vi "NV measurements.vi"(0 "Number of samples":dbl=50000.0, 1 "Pulse mode":T1(ring), 2 "Initial duration (ns)":dbl=1.0 format="%#_13g", 3 "Final duration (ns)":dbl=1.0 format="%#_13g", 4 "AOM on":dbl[unit]=9.999999999999999e-06 format="%#_13p", 5 "AOM off":dbl[unit]=9.999999999999999e-05 format="%#_13p", 6 "N type output level value (-136dBm to 0 dBm)":dbl=-20.0, 7 "Duration increment (ns)":dbl=1.0 format="%#_13g", 8 "file (use dialog)":path=path "C:/Users/Choi group/Dropbox/Labbook/Quantum Optics/hBN/230726/attoDRY", 9 "pi":dbl[unit] format="%#_13p", 10 "Initial frequency (MHz)":dbl=1500.0 format="%#_13g", 11 "pi/2":dbl[unit] format="%#_13p", 12 "Final frequency (MHz)":dbl=2500.0 format="%#_13g", 13 "Contrast calculation":T3(ring), 14 "Frequency increment (MHz)":dbl=10.0 format="%#_13g", 15 "Modulation type":u16(ring)=4 items=["AM/ASK"=0, "FM/FSK"=1, "PM/PSK"=2, "Sweep"=3, "Pulse"=4, "Blank"=5, "QAM"=7, "CPM"=8, "VSB"=9], 16 "Measurement #":i32=11, 18 "Averaging?":bool, 19 "Parameters logging?":bool=TRUE) -> ()   [LabVIEW 2015]
uses:
  Libraries/Stanford Research SG39x Series/Stanford Research SG39x Series.lvlib
  <vilib>/Utility/file.llb/Write Delimited Spreadsheet (string).vi
  Libraries/SR400/Public/Typedefs/Output Scale.ctl
  Libraries/SR400/SR400.lvlib
panel:
  in  "file path for measurement parameters":path=path "C:/Users/Choi group/Dropbox/Labbook/Quantum Optics/hBN/230726/attoDRY/parameters log.txt"
  out "file?":bool
  in  "Tab Control":T2(tab)=enum."AFG3252"
  in  "VISA_SG396":refnum<visa-resource-name>="GPIB0::27::INSTR"
  in  "Location of spinapi.dll":path=path "C:/SpinCore/SpinAPI/lib/spinapi64.dll"
  in  "pi_Y":dbl[unit] format="%#_13p"
  in  "VISA_SR400_1":refnum<visa-resource-name>="GPIB0::18::INSTR"
  in  "VISA_SR400_2":refnum<visa-resource-name>="GPIB0::18::INSTR"
  in  "Gate A width":dbl[unit]=8.000000000000001e-06
  in  "Gate A delay":dbl[unit]=2.0000000000000003e-06
  in  "Gate B width":dbl[unit]=8.000000000000001e-06
  in  "Gate B delay":dbl[unit]=2.0000000000000003e-06
  in  "Gate delay offset":dbl[unit]=7.000000000000001e-09
  in  "Gate width offset":dbl[unit]=8e-09
  in  "Gain":dbl=0.6
  in  "margin (ns)":i32=20
  in  "resolution (ns)":dbl=0.5 format="%#_13g"
  in  "AFG to MW switch delay":dbl[unit]=2.3000000000000002e-07 format="%#_13g"
  in  "N of XY8-N":i32=1
  in  "MW switch margin (ns)":dbl=30.0 format="%#_13g"
  out "Current frequency (MHz)":dbl=2980.0 format="%#.9f"
  out "Contrast":dbl=0.9066760283189983
  out "Sig1_temp":dbl=15496.0
  out "Sig2_temp":dbl=17091.0
  out "Ref1_temp":dbl=15202.0
  out "Ref2_temp":dbl=17166.0
  out "Iteration":i32=1662
  out "Current duration":dbl[unit]
  out "Averaged counts":dbl=0.9066760283189983
  out "XY Graph":cluster{"Y":dbl[], "Y":dbl[]}[](graph)=[{"Y"=[10.0, 12.0, 14.0, 16.0, 18.0, 20.0, 22.0, 24.0, 26.0, 28.0, 30.0, 32.0, 34.0, 36.0, 38.0, 40.0, 42.0, 44.0, 46.0, 48.0, 50.0, 52.0, 54.0, 56.0, 58.0, 60.0, 62.0, 64.0, 66.0, 68.0, 70.0, 72.0, 74.0, 76.0, 78.0, 80.0, 82.0, 84.0, 86.0, 88.0, 90.0, 92.0, 94.0, 96.0, 98.0, 100.0], "Y"=[0.8767203858369602, 0.8691455977263308, 0.8745225141798818, 0.9030268088786394, 0.9378455450154222, 0.9275370747310265, 0.9308731504766361, 0.9057829759584146, 0.8666319504715616, 0.8803564101061023, 0.906591799730947, 0.9180885370858985, 0.9439413797211962, 0.9016052661970204, 0.8839480638860162, 0.8758135750813575, 0.8816878889967453, 0.913326362263274, 0.9088317463937511, 0.9162288551469315, 0.9055664853604907, 0.9089218250508573, 0.8930382664822499, 0.8875780707841776, 0.9212244897959184, 0.9054543364561183, 0.8933922728055571, 0.9381969714755253, 0.8942631517826036, 0.8838066088533696, 0.8963005448809865, 0.9031774407473616, 0.9180577520060914, 0.9075721912853779, 0.8828040674884963, 0.90195394277739, 0.8791781135531136, 0.9186380980334605, 0.9048862581244196, 0.9063314603487227, 0.9013971137814063, 0.8959866605335787, 0.9040195451108138, 0.8972309118294519, 0.9009098914000586, 0.9066760283189983]}]
  out "XY Graph 2":cluster{"Y":dbl[], "Y":dbl[]}[](graph)=[{"Y"=[2980.0], "Y"=[0.8767203858369602]}]
  in  "stop":bool
  out "file":refnum<file>
  # "IQ modulation ON: QAM\nIQ modulation OFF: Pulse"
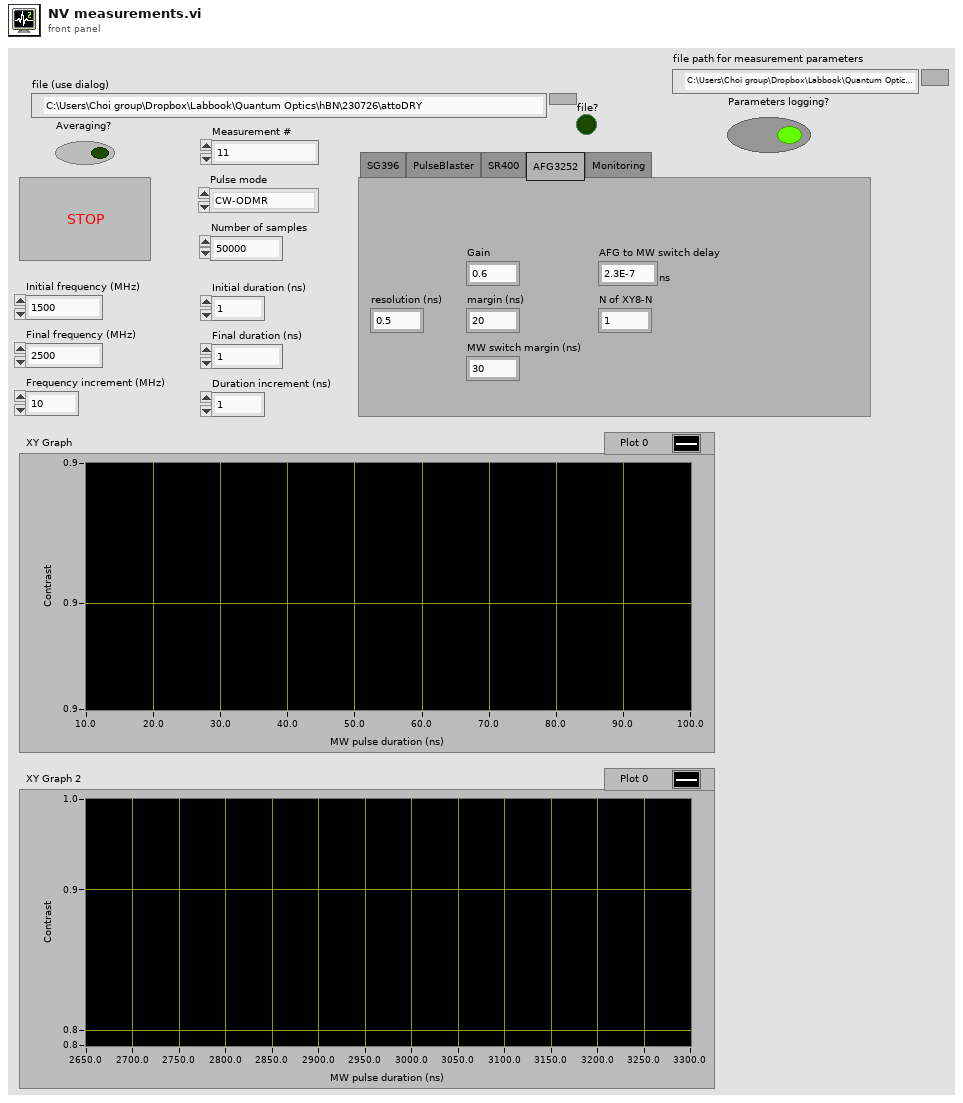
[diagram p1: front panel]
types:
  T1 = enum16{"CW-ODMR", "Rabi", "Rabi_IQ", "Ramsey", "Spin echo decay", "Spin echo_IQ", "CPMG", "XY4", "XY8", "XY8-N", "Corr-XY8", "T1 relaxation", "T1_IQ"}
  T2 = enum32{"SG396", "PulseBlaster", "SR400", "AFG3252", "Monitoring"}
  T3 = enum16{"sig1/sig2", "sig1/ref2", "(sig2-sig1)/(sig2+sig1)", "(sig2-sig1)/ref1"}
  T4 = enum16{"open", "replace", "create", "open or create", "replace or create", "replace or create with confirmation"}
  T5 = typedef "SR400.lvlib/Output Scale.ctl" = enum16{"Log", "987######", "#876#####", "##765####", "###654###", "####543##", "#####432#", "######321"}
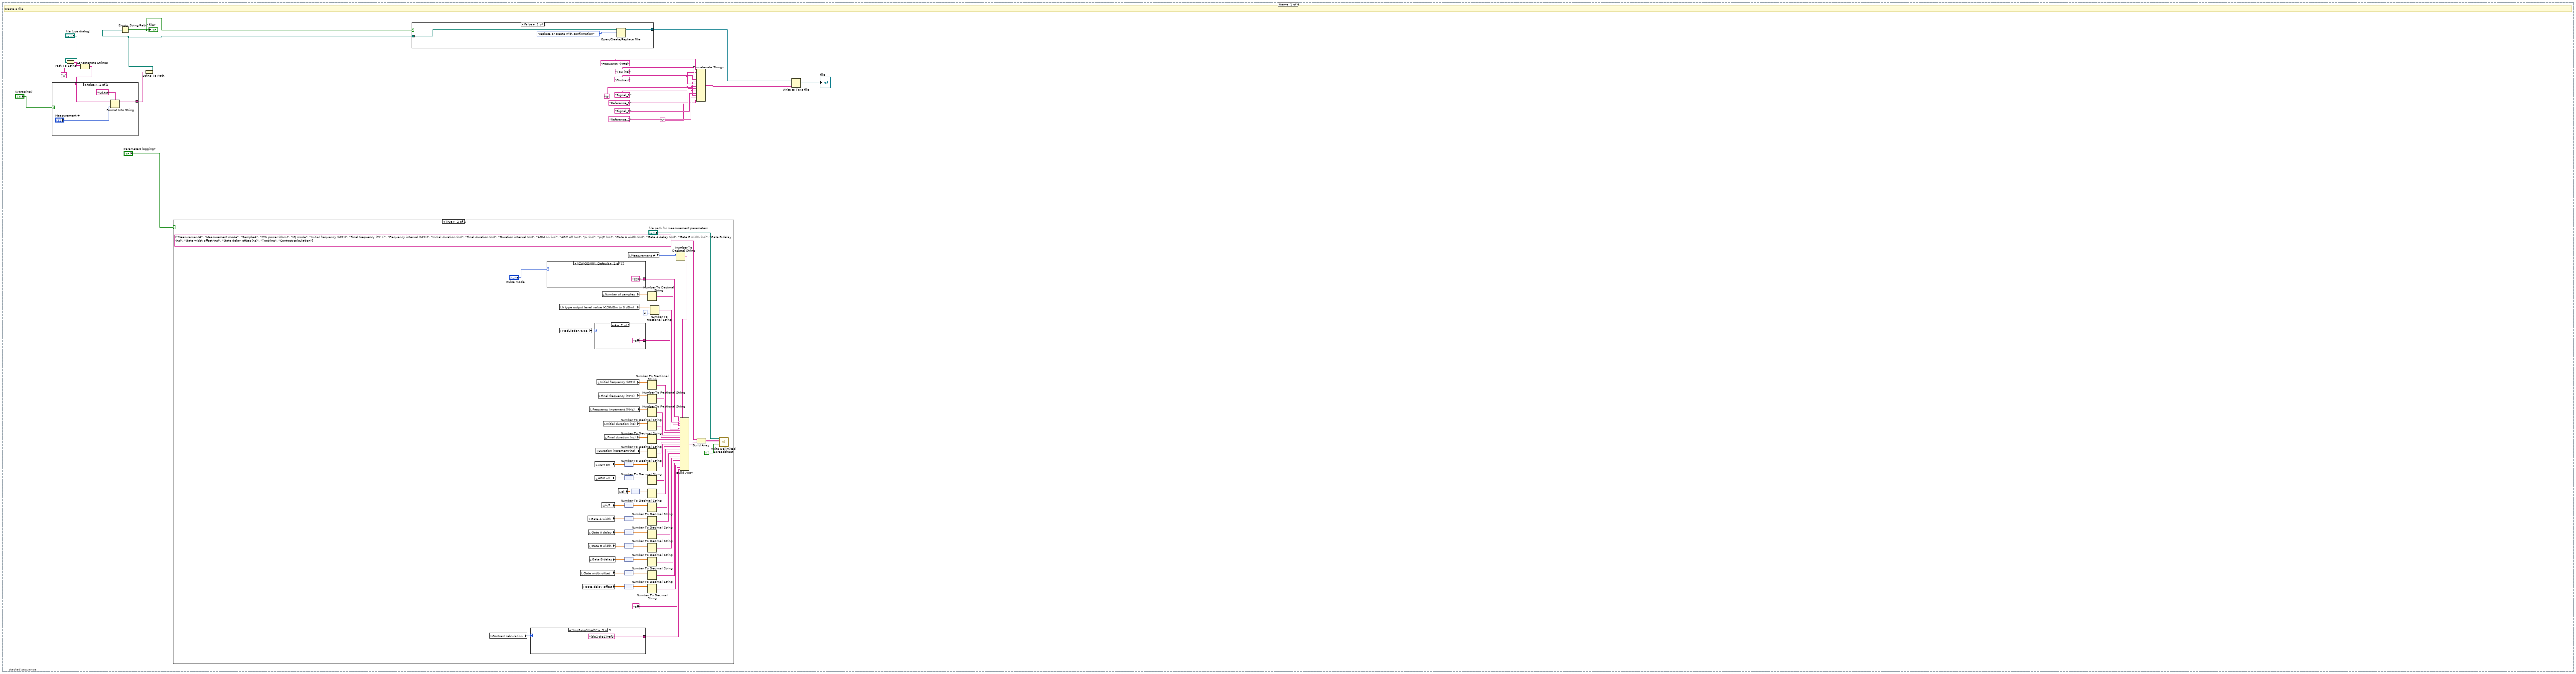
[diagram p2: hidden frame]
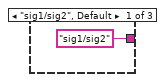
[diagram p5: hidden frame]
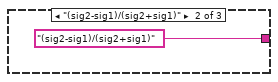
[diagram p6: hidden frame]
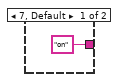
[diagram p7: hidden frame]
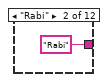
[diagram p8: hidden frame]
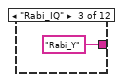
[diagram p9: hidden frame]
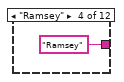
[diagram p10: hidden frame]
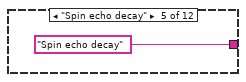
[diagram p11: hidden frame]
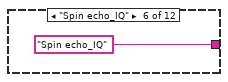
[diagram p12: hidden frame]
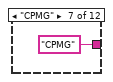
[diagram p13: hidden frame]
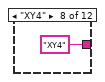
[diagram p14: hidden frame]
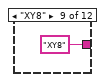
[diagram p15: hidden frame]
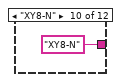
[diagram p16: hidden frame]
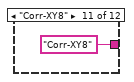
[diagram p17: hidden frame]
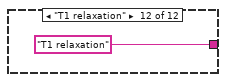
[diagram p18: hidden frame]
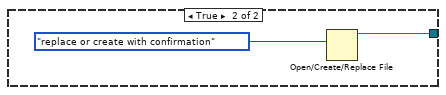
[diagram p19: hidden frame]
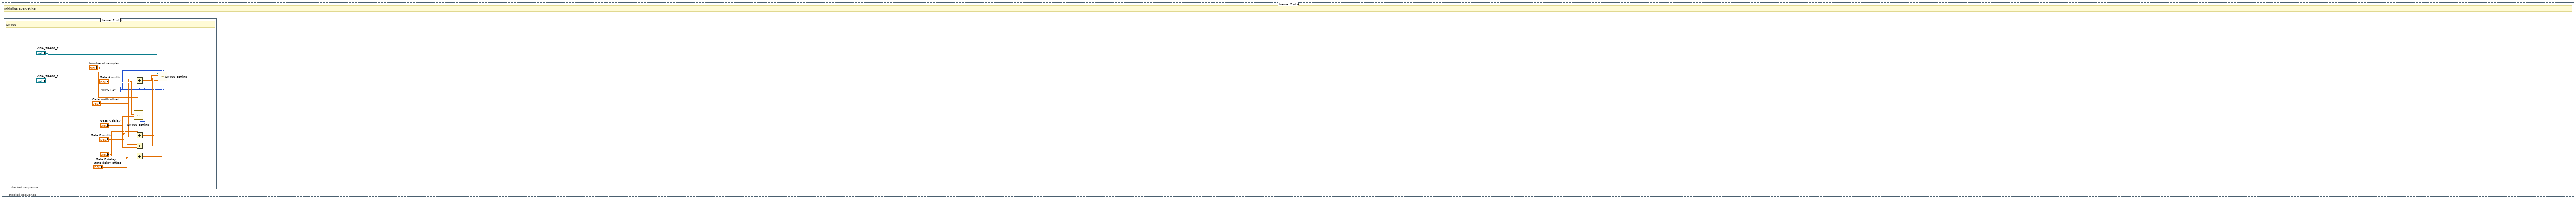
[diagram p20: hidden frame]
diagram:
  n1 = stacked-sequence {
    frame #0 {
      w1 = "\t"
      # "Create a file"
      n2 = Path To String(path="file (use dialog)") -> (string=w6:string)
      n3 = Concatenate Strings(w6, "\\" ("string")) -> (w4:string)
      n4 = case shown="False" "Averaging?" {
        tunnel: w4 -> [w23 w26]
        tunnel: [w24 w26] -> w7
        frame False {
          n5 = Format Into String(format string="%d.txt", initial string=w23, "Measurement #") -> (resulting string=w24:string)  [unwired: 1 in, 1 out]
        }
        frame True {
        }
      }
      n6 = String To Path(string=w7) -> (path=w3:path)
      n7 = Empty String/Path?(string/path=w3) -> (empty?=w21:bool)
      "file?" <- w21
      n8 = case shown="True" "Parameters logging?" {
        frame False {
        }
        frame True {
          n9 = local read "Contrast calculation"() -> (w35:T3)
          n10 = case shown="\"(sig2-sig1)/ref1\"" w35 {
            tunnel: ["sig1/sig2" "(sig2-sig1)/(sig2+sig1)" "(sig2-sig1)/ref1"] -> w34
            frame "sig1/sig2", Default {
            }
            frame "(sig2-sig1)/(sig2+sig1)" {
            }
            frame "(sig2-sig1)/ref1" {
            }
          }
          n11 = case shown="\"CW-ODMR\", Default" "Pulse mode" {
            tunnel: ["ESR" "Rabi" "Rabi_Y" "Ramsey" "Spin echo decay" "Spin echo_IQ" "CPMG" "XY4" "XY8" "XY8-N" "Corr-XY8" "T1 relaxation"] -> w30
            frame "CW-ODMR", Default {
            }
            frame "Rabi" {
            }
            frame "Rabi_IQ" {
            }
            frame "Ramsey" {
            }
            frame "Spin echo decay" {
            }
            frame "Spin echo_IQ" {
            }
            frame "CPMG" {
            }
            frame "XY4" {
            }
            frame "XY8" {
            }
            frame "XY8-N" {
            }
            frame "Corr-XY8" {
            }
            frame "T1 relaxation" {
            }
          }
          n12 = local read "N type output level value (-136dBm to 0 dBm)"() -> (w86:dbl)
          n13 = local read "Modulation type"() -> (w84:u16)
          n14 = local read "Gate width offset"() -> (w57:dbl[unit])
          n15 = local read "Gate delay offset"() -> (w56:dbl[unit])
          n16 = local read "Gate A width"() -> (w61:dbl[unit])
          n17 = local read "Gate A delay"() -> (w60:dbl[unit])
          n18 = local read "Gate B width"() -> (w59:dbl[unit])
          n19 = local read "Gate B delay"() -> (w58:dbl[unit])
          n20 = local read "Frequency increment (MHz)"() -> (w81:dbl)
          n21 = case shown="4" w84 {
            tunnel: ["on" "off"] -> w33
            frame 7, Default {
            }
            frame 4 {
            }
          }
          n22 = local read "AOM on"() -> (w71:dbl[unit])
          n23 = local read "AOM off"() -> (w70:dbl[unit])
          n24 = local read "Duration increment (ns)"() -> (w72:dbl)
          n25 = local read "Initial frequency (MHz)"() -> (w83:dbl)
          n26 = local read "Final frequency (MHz)"() -> (w82:dbl)
          n27 = local read "pi/2"() -> (w62:dbl[unit])
          n28 = local read "Number of samples"() -> (w87:dbl)
          n29 = local read "Initial duration (ns)"() -> (w74:dbl)
          n30 = local read "Final duration (ns)"() -> (w73:dbl)
          n31 = local read "pi"() -> (w63:dbl[unit])
          n32 = node(w71) -> (w69:dbl)
          n33 = node(w70) -> (w68:dbl)
          n34 = node(w62) -> (w54:dbl)
          n35 = node(w61) -> (w53:dbl)
          n36 = node(w60) -> (w52:dbl)
          n37 = node(w59) -> (w51:dbl)
          n38 = node(w58) -> (w50:dbl)
          n39 = node(w57) -> (w49:dbl)
          n40 = node(w56) -> (w48:dbl)
          n41 = local read "Measurement #"() -> (w29:i32)
          n42 = node(w63) -> (w55:dbl)
          n43 = Number To Decimal String(number=w87) -> (decimal integer string=w31:string)  [unwired: 1 in]
          n44 = Number To Fractional String(number=w83) -> (F-format string=w80:string)  [unwired: 3 in]
          n45 = Number To Fractional String(number=w82) -> (F-format string=w79:string)  [unwired: 3 in]
          n46 = Number To Fractional String(number=w81) -> (F-format string=w78:string)  [unwired: 3 in]
          n47 = Number To Decimal String(number=w74) -> (decimal integer string=w77:string)  [unwired: 1 in]
          n48 = Number To Decimal String(number=w73) -> (decimal integer string=w76:string)  [unwired: 1 in]
          n49 = Number To Decimal String(number=w72) -> (decimal integer string=w75:string)  [unwired: 1 in]
          n50 = Number To Decimal String(number=w69) -> (decimal integer string=w67:string)  [unwired: 1 in]
          n51 = Number To Decimal String(number=w68) -> (decimal integer string=w66:string)  [unwired: 1 in]
          n52 = Number To Decimal String(number=w55) -> (decimal integer string=w65:string)  [unwired: 1 in]
          n53 = Number To Decimal String(number=w54) -> (decimal integer string=w64:string)  [unwired: 1 in]
          n54 = Number To Decimal String(number=w53) -> (decimal integer string=w47:string)  [unwired: 1 in]
          n55 = Number To Decimal String(number=w52) -> (decimal integer string=w46:string)  [unwired: 1 in]
          n56 = Number To Decimal String(number=w51) -> (decimal integer string=w45:string)  [unwired: 1 in]
          n57 = Number To Decimal String(number=w50) -> (decimal integer string=w44:string)  [unwired: 1 in]
          n58 = Number To Decimal String(number=w49) -> (decimal integer string=w43:string)  [unwired: 1 in]
          n59 = Number To Decimal String(number=w48) -> (decimal integer string=w42:string)  [unwired: 1 in]
          n60 = Number To Fractional String(number=w86, precision (6)=i16 2) -> (F-format string=w32:string)  [unwired: 2 in]
          n61 = Number To Decimal String(number=w29) -> (decimal integer string=w28:string)  [unwired: 1 in]
          n62 = Build Array(w28, w30, w31, w32, w33, w80, w79, w78, w77, w76, w75, w67, w66, w65, w64, w47, w46, w45, w44, w43, w42, "off", w34) -> (w39:string[])
          n63 = Build Array(string[] ["Measurement#", "Measurement mode", "Sample#", "MW power (dbm)", "IQ mode", "Initial frequency (MHz)", "Final frequency (MHz)", "Frequency interval (MHz)", "Initial duration (ns)", "Final duration (ns)", "Duration interval (ns)", "AOM on (us)", "AOM off (us)", "pi (ns)", "pi/2 (ns)", "Gate A width (ns)", "Gate A delay (ns)", "Gate B width (ns)", "Gate B delay (ns)", "Gate width offset (ns)", "Gate delay offset (ns)", "Tracking", "Contrast calculation"] ("Parameters list"), w39) -> (w36:string[][])
          n64 = call-poly <vilib>:"Write Delimited Spreadsheet.vi"("file path (dialog if empty)"="file path for measurement parameters", "2D data"=w36, "append to file? (F)"=TRUE) -> ()  [unwired: 11 in, 2 out]
        }
      }
      n65 = case shown="False" w21 {
        tunnel: w3 -> [w106 _]
        tunnel: [w105 w108] -> w14
        frame False {
          n66 = Open/Create/Replace File(file path (use dialog)=w106, operation (0:open)=T4."replace or create with confirmation") -> (refnum out=w105:refnum<file>)  [unwired: 4 in, 2 out]
        }
        frame True {
          n67 = Open/Create/Replace File(operation (0:open)=T4."replace or create with confirmation") -> (refnum out=w108:refnum<file>)  [unwired: 5 in, 2 out]
        }
      }
      n68 = Concatenate Strings("Frequency (MHz)" ("string"), w1, "Tau (ns)" ("string"), w1, "Contrast" ("string"), w1, "Signal_1" ("string"), w1, "Reference_1" ("string"), w1, "Signal_2" ("string"), w1, "Reference_2" ("string"), "\r") -> (w16:string)
      n69 = Write to Text File(file (use dialog)=w14, text=w16) -> (refnum out=→"file":refnum<file>)  [unwired: 2 in, 2 out]
    }
    frame #1 {
      # "Initialize everything"
      n70 = stacked-sequence {
        frame #0 {
          # "Microwave"
          n71 = local read "Initial frequency (MHz)"() -> (w115:dbl)
          n72 = case shown="7" "Modulation type" {
            tunnel: [FALSE ("BNC output") TRUE ("N type output")] -> w110
            frame 4, Default {
            }
            frame 7 {
            }
          }
          n73 = call "Initialize.vi"("VISA resource name"="VISA_SG396") -> ("VISA resource name out"=w113:refnum<visa-resource-name>)  [unwired: 9 in, 1 out]
          n74 = call "Set_SG394_Frequency.vi"("Frequency (MHz)"=w115, "VISA resource name"=w113) -> ("VISA resource name out"=w112:refnum<visa-resource-name>)  [unwired: 1 in, 1 out]
          n75 = call "Set_SG394_Mode.vi"("Modulation type"="Modulation type", "Modulation"=w110, "N type Amplitude (-110 to 0 dBm)"="N type output level value (-136dBm to 0 dBm)", "N type output"=TRUE, "BNC output"=FALSE, "VISA resource name"=w112) -> ()  [unwired: 4 in, 2 out]
        }
        frame #1 {
          w123 = enum16{"10 MHz", "INPUT 1", "INPUT 2", "TRIG"}."INPUT 1" ("Counter A Input")
          # "SR400"
          n76 = call "SR400_setting.vi"("Counter B Input"=w123, "Counter A Input"=w123, "Gate B delay"="Gate B delay", "Number of samples"="Number of samples", "Gate B width"="Gate B width", "Gate A delay"="Gate A delay", "Gate A width"="Gate A width", "VISA_SR400"="VISA_SR400_1") -> ()  [unwired: 4 in]
          n77 = Add(x="Gate width offset", y="Gate A width") -> (x+y=w130:dbl[unit])
          n78 = Add(x="Gate B width", y="Gate width offset") -> (x+y=w127:dbl[unit])
          n79 = Add(x="Gate delay offset", y="Gate A delay") -> (x+y=w131:dbl[unit])
          n80 = Add(x="Gate B delay", y="Gate delay offset") -> (x+y=w126:dbl[unit])
          n81 = call "SR400_setting.vi"("Counter B Input"=w123, "Counter A Input"=w123, "Gate B delay"=w126, "Number of samples"="Number of samples", "Gate B width"=w127, "Gate A delay"=w131, "Gate A width"=w130, "VISA_SR400"="VISA_SR400_2") -> ()  [unwired: 4 in]
        }
        frame #2 {
          # "AFG3252"
        }
      }
    }
    frame #2 {
      w135 = dbl[] []  # Freq array for plot
      w136 = dbl[] []  # Contrast array for plot
      # "Measurement"
      n82 = Subtract(x="Final frequency (MHz)", y="Initial frequency (MHz)") -> (x-y=w143:dbl)
      n83 = Divide(x=w143, y="Frequency increment (MHz)") -> (x/y=w142:dbl)
      n84 = To Unsigned Long Integer(number=w142) -> (unsigned 32bit integer=w139:u32)
      n85 = while {
        tunnel: "Frequency increment (MHz)" -> [w154]
        tunnel: w139 -> [w158]
        shift-right: [w153] -> _
        shift-left: "Initial frequency (MHz)" -> [w160]
        tunnel: "Initial duration (ns)" -> [w152]
        tunnel: "Duration increment (ns)" -> [w151]
        shift-right: [w145] -> _
        shift-left: w136 -> [w149]
        shift-right: [w147] -> _
        shift-left: w135 -> [w148]
        i -> [w159]
        stop <- w155 stop-if-true
        n86 = flat-sequence {
          tunnel: w160 -> [w161]
          tunnel: w154 -> [w166]
          tunnel: [w165] -> w153
          tunnel: [w161] -> w150
          tunnel: w149 -> [w164]
          tunnel: [w163] -> w145
          tunnel: w152 -> [w175]
          tunnel: w151 -> [w174]
          tunnel: w150 -> [w173]
          tunnel: w148 -> [w169]
          tunnel: [w167] -> w146
          tunnel: [w436] -> w147
          tunnel: w146 -> [w436]
          tunnel: w145 -> [w438]
          frame #0 {
            # "Change MW frequency"
            n87 = Add(x=w161, y=w166) -> (x+y=w165:dbl)
            n88 = Build Array (concatenate)(w164, w161) -> (w163:dbl[])
            n89 = local read "VISA_SG396"() -> (w162:refnum<visa-resource-name>)
            n90 = call "Set_SG394_Frequency.vi"("Frequency (MHz)"=w161, "VISA resource name"=w162) -> ()  [unwired: 1 in, 2 out]
            "Current frequency (MHz)" <- w161
          }
          frame #1 {
            w171 = dbl[] []  # Duration array for plot
            w172 = dbl[] []  # Contrast array for plot 2
            # "Measure"
            n91 = while {
              shift-right: [w186] -> _
              shift-left: w175 -> [w179]
              tunnel: w174 -> [w185]
              tunnel: w173 -> [w184]
              shift-right: [w182] -> w170
              shift-left: w172 -> [w183]
              shift-right: [w180] -> _
              shift-left: w171 -> [w181]
              i -> [w177]
              stop <- w187 stop-if-true
              n92 = Increment(x=w177) -> (x+1=w176:i32)
              n93 = stacked-sequence {
                seq-local: [_ w289 _] -> [_ _ w382]
                seq-local: [_ w290 _] -> [_ _ w380]
                seq-local: [w206 _ _] -> [_ w280 _]
                seq-local: [_ w273 _] -> [_ _ w381]
                seq-local: [_ w272 _] -> [_ _ w371]
                tunnel: w179 -> [w193 _ w377]
                tunnel: [w198 _ _] -> w186
                tunnel: w185 -> [w192 _ _]
                tunnel: w184 -> [_ _ w390]
                tunnel: w183 -> [_ _ w396]
                tunnel: [_ _ w392] -> w182
                tunnel: w181 -> [_ _ w395]
                tunnel: [_ _ w376] -> w180
                tunnel: w176 -> [w194 _ _]
                frame #0 {
                  # "Set pulse sequence"
                  n94 = node(w193) -> (w202:dbl[unit])
                  "Current duration" <- w202
                  n95 = local read "Pulse mode"() -> (w190:T1)
                  n96 = case shown="\"T1_IQ\"" w190 {
                    tunnel: w194 -> [_ w214]
                    tunnel: w192 -> [w208 w213]
                    tunnel: [w208 w209] -> w191
                    frame "CW-ODMR", Default {
                      # "equal interval"
                    }
                    frame "T1_IQ" {
                      # "non-equal interval"
                      n97 = Multiply(x=w213, y=w214) -> (x*y=w215:dbl)
                      n98 = Power Of X(1:w215, 2:1.15 ("y")) -> (0:w217:dbl)
                      n99 = Multiply(x=w217, y=0.1) -> (x*y=w212:dbl)
                      n100 = Round To Nearest(number=w212) -> (nearest integer value=w211:dbl)
                      n101 = Quotient & Remainder(x=w211, y=100.0) -> (x-y*floor(x/y)=w210:dbl)  [unwired: 1 out]
                      n102 = Subtract(x=w211, y=w210) -> (x-y=w209:dbl)
                    }
                  }
                  n103 = case shown="\"Rabi_IQ\"" w190 {
                    tunnel: [w220 w221 w224 w229 w238 w243 w244 w252 w253 w254 w255 w256 w271] -> w201
                    tunnel: w202 -> [w220 w221 w224 w229 w238 w243 w244 w252 w253 w254 w255 w256 w271]
                    tunnel: [_ _ _ _ _ _ _ _ _ _ _ w257 _] -> w195
                    frame "CW-ODMR", Default {
                    }
                    frame "Rabi" {
                    }
                    frame "Rabi_IQ" {
                      n104 = local read item#-1() -> (w228)
                      n105 = local read "resolution (ns)"() -> (w223:dbl)
                      n106 = call "Rabi.vi"("Gain"="Gain", "resolution (ns)"=w223, "margin (ns)"="margin (ns)", "Pi pulse duration"=w224) -> ("Array size"=w222:dbl, "Array"=w226:dbl[])  [unwired: 6 in]
                      n107 = call "Set AFG3252 pulse sequence.vi"("Channel 2"=w226, "Array size"=w222, "Channel 1"=w226, "Gain (1 V)"="Gain", "VISA resource name"=w228) -> ()  [unwired: 7 in]
                    }
                    frame "Spin echo decay" {
                    }
                    frame "Spin echo_IQ" {
                      n108 = local read "MW switch margin (ns)"() -> (w232:dbl)
                      n109 = local read "resolution (ns)"() -> (w231:dbl)
                      n110 = local read "margin (ns)"() -> (w233:i32)
                      n111 = local read "AOM on"() -> (w237:dbl[unit])
                      n112 = local read "AOM off"() -> (w236:dbl[unit])
                      n113 = local read "Gain"() -> (w241:dbl)
                      n114 = local read "pi/2"() -> (w239:dbl[unit])
                      n115 = local read "pi"() -> (w240:dbl[unit])
                      n116 = local read item#-1() -> (w242)
                      n117 = call "Spin echo.vi"("Free precession time"=w238, "MW switch margin (ns)"=w232, "resolution (ns)"=w231, "margin (ns)"=w233, "Gain"=w241, "pi"=w240, "AOM on"=w237, "AOM off"=w236, "pi/2"=w239) -> ("Array size"=w230:i32, "I"=w235:dbl[], "Q"=w234:dbl[])  [unwired: 4 in]
                      n118 = call "Set AFG3252 pulse sequence.vi"("Channel 2"=w234, "Array size"=w230, "Channel 1"=w235, "Gain (1 V)"=w241, "VISA resource name"=w242) -> ()  [unwired: 7 in]
                    }
                    frame "Ramsey" {
                    }
                    frame "T1 relaxation" {
                    }
                    frame "T1_IQ" {
                      n119 = local read "resolution (ns)"() -> (w247:dbl)
                      n120 = local read "margin (ns)"() -> (w248:i32)
                      n121 = local read "Gain"() -> (w250:dbl)
                      n122 = local read "pi"() -> (w249:dbl[unit])
                      n123 = local read item#-1() -> (w251)
                      n124 = call "T1.vi"("resolution (ns)"=w247, "pi"=w249, "Gain"=w250, "margin (ns)"=w248) -> ("Array"=w246:dbl[], "Array size"=w245:i32)  [unwired: 6 in]
                      n125 = call "Set AFG3252 pulse sequence.vi"("Channel 2"=w246, "Array size"=w245, "Channel 1"=w246, "Gain (1 V)"=w250, "VISA resource name"=w251) -> ()  [unwired: 7 in]
                    }
                    frame "CPMG" {
                    }
                    frame "XY4" {
                    }
                    frame "XY8" {
                    }
                    frame "XY8-N" {
                      n126 = local read "MW switch margin (ns)"() -> (w265:dbl)
                      n127 = local read "margin (ns)"() -> (w261:i32)
                      n128 = local read "AOM on"() -> (w260:dbl[unit])
                      n129 = local read "AOM off"() -> (w259:dbl[unit])
                      n130 = local read "Gain"() -> (w266:dbl)
                      n131 = local read "pi/2"() -> (w262:dbl[unit])
                      n132 = local read "pi"() -> (w263:dbl[unit])
                      n133 = local read item#-1() -> (w270)
                      n134 = call "XY8-N.vi"("Tau"=w256, "Gain"=w266, "MW switch margin (ns)"=w265, "resolution (ns)"="resolution (ns)", "pi"=w263, "pi/2"=w262, "margin (ns)"=w261, "AOM on"=w260, "AOM off"=w259, "N"="N of XY8-N") -> ("Array size"=w269:dbl, "I array"=w268:dbl[], "Q array"=w267:dbl[], "pulse length (ns)"=w257:dbl)  [unwired: 2 in]
                      n135 = call "Set AFG3252 pulse sequence.vi"("Channel 2"=w267, "Array size"=w269, "Channel 1"=w268, "Gain (1 V)"=w266, "VISA resource name"=w270) -> ()  [unwired: 7 in]
                    }
                    frame "Corr-XY8" {
                    }
                  }
                  n136 = local read "Location of spinapi.dll"() -> (w207:path)
                  n137 = Add(x=w193, y=w191) -> (x+y=w198:dbl)
                  n138 = call "20230426_sequence_setting_ShortPulseFeature.vi"("AOM on"="AOM on", "AOM off"="AOM off", "sweeping t"=w201, "pi"="pi", "pi/2"="pi/2", "pi_Y"="pi_Y", "Path"=w207, "Pulse mode"=w190, "pulse length (ns)"=w195, "AFG to MW switch delay"="AFG to MW switch delay", "MW switch margin (ns)"="MW switch margin (ns)") -> ("path out"=w206:path)  [unwired: 8 in]
                }
                frame #1 {
                  # "Extract signals"
                  n139 = flat-sequence {
                    tunnel: [w295] -> w287
                    tunnel: [w294] -> w285
                    tunnel: [w293] -> w283
                    tunnel: [w292] -> w281
                    tunnel: [w309] -> w288
                    tunnel: w287 -> [w309]
                    tunnel: [w308] -> w286
                    tunnel: w285 -> [w308]
                    tunnel: [w307] -> w284
                    tunnel: w283 -> [w307]
                    tunnel: [w306] -> w282
                    tunnel: w281 -> [w306]
                    tunnel: w280 -> [w305]
                    tunnel: [w304] -> w278
                    tunnel: w288 -> [w318]
                    tunnel: w286 -> [w317]
                    tunnel: w284 -> [w316]
                    tunnel: w282 -> [w315]
                    tunnel: [w314] -> w279
                    tunnel: w278 -> [w314]
                    tunnel: [w313] -> w277
                    tunnel: [w312] -> w276
                    tunnel: [w311] -> w275
                    tunnel: [w310] -> w274
                    tunnel: [w363] -> w289
                    tunnel: [w364] -> w290
                    tunnel: w279 -> [w370]
                    tunnel: w277 -> [w366]
                    tunnel: w276 -> [w365]
                    tunnel: w275 -> [w362]
                    tunnel: w274 -> [w360]
                    tunnel: [w356] -> w273
                    tunnel: [w355] -> w272
                    frame #0 {
                      n140 = Wait (ms)(milliseconds to wait=u32 100) -> ()  [unwired: 1 out]
                      n141 = local read "VISA_SR400_1"() -> (w298:refnum<visa-resource-name>)
                      n142 = local read "VISA_SR400_2"() -> (w301:refnum<visa-resource-name>)
                      n143 = String Subset(string=w298, offset (0)=7, length (rest)=2 ("length (rest)")) -> (substring=w294:string)
                      n144 = String Subset(string=w301, offset (0)=7, length (rest)=2 ("length (rest)")) -> (substring=w295:string)
                      n145 = GPIB Write(0:w294, 1:"CR; CS;" ("data")) -> (6:w293:errorcluster)  [unwired: 3 in, 1 out]
                      n146 = GPIB Write(0:w295, 1:"CR; CS;" ("data")) -> (6:w292:errorcluster)  [unwired: 3 in, 1 out]
                    }
                    frame #1 {
                      n147 = call "Start_PulseBlaster.vi"("path in"=w305) -> ("path out"=w304:path)
                    }
                    frame #2 {
                      n148 = while {
                        tunnel: w317 -> [w331]
                        tunnel: w316 -> [w345]
                        tunnel: [w320] -> w313
                        tunnel: w318 -> [w333]
                        tunnel: w315 -> [w340]
                        tunnel: [w322] -> w312
                        tunnel: [w321] -> w311
                        tunnel: [w323] -> w310
                        i -> [w350]
                        stop <- w337 continue-if-true
                        w319 = 0.0 ("y")
                        n149 = GPIB Write(0:w331, 1:"QA1; QB1" ("data string"), 3:w345) -> (6:w348:errorcluster)  [unwired: 2 in, 1 out]
                        n150 = GPIB Write(0:w333, 1:"QA1; QB1" ("data string"), 3:w340) -> (6:w342:errorcluster)  [unwired: 2 in, 1 out]
                        n151 = GPIB Read(0:w331, 1:20 ("byte count"), 3:w348) -> (5:w347:string, 7:w332:errorcluster)  [unwired: 2 in, 1 out]
                        n152 = GPIB Read(0:w333, 1:20 ("byte count"), 3:w342) -> (5:w343:string, 7:w334:errorcluster)  [unwired: 2 in, 1 out]
                        n153 = Fract/Exp String To Number(string=w347) -> (number=w320:dbl)  [unwired: 3 in, 1 out]
                        "Sig1_temp" <- w320
                        n154 = Fract/Exp String To Number(string=w343) -> (number=w321:dbl)  [unwired: 3 in, 1 out]
                        "Sig2_temp" <- w321
                        n155 = GPIB Read(0:w331, 1:20 ("byte count"), 3:w332) -> (5:w330:string)  [unwired: 2 in, 2 out]
                        n156 = GPIB Read(0:w333, 1:20 ("byte count"), 3:w334) -> (5:w329:string)  [unwired: 2 in, 2 out]
                        n157 = Fract/Exp String To Number(string=w330) -> (number=w322:dbl)  [unwired: 3 in, 1 out]
                        "Ref1_temp" <- w322
                        n158 = Fract/Exp String To Number(string=w329) -> (number=w323:dbl)  [unwired: 3 in, 1 out]
                        "Ref2_temp" <- w323
                        n159 = local read "stop"() -> (w339:bool)
                        n160 = Greater?(x=w319, y=w322) -> (0:w327:bool)
                        n161 = Greater?(x=w319, y=w321) -> (0:w326:bool)
                        n162 = Greater?(x=w319, y=w320) -> (0:w325:bool)
                        n163 = Greater?(x=w319, y=w323) -> (0:w328:bool)
                        n164 = Not(x=w339) -> (.not. x?=w338:bool)
                        n165 = Compound Arithmetic op=OR(w325, w326, w327, w328) -> (w324:bool)
                        n166 = And(x=w338, y=w324) -> (x .and. y?=w337:bool)
                        "Iteration" <- w350
                      }
                    }
                    frame #3 {
                      n167 = call "Stop_PulseBlaster.vi"("path in"=w370) -> ()  [unwired: 1 out]
                      n168 = local read "Gate B width"() -> (w354:dbl[unit])
                      n169 = local read "Gate A width"() -> (w367:dbl[unit])
                      n170 = node(w354) -> (w353:dbl)
                      n171 = node(w367) -> (w358:dbl)
                      n172 = local read "Number of samples"() -> (w357:dbl)
                      n173 = Divide(x=w365, y=w353) -> (x/y=w369:dbl)
                      n174 = Divide(x=w362, y=w358) -> (x/y=w361:dbl)
                      n175 = Divide(x=w360, y=w353) -> (x/y=w359:dbl)
                      n176 = Divide(x=w366, y=w358) -> (x/y=w368:dbl)
                      n177 = local read item#-1() -> (w351)
                      n178 = VISA Write(VISA resource name=w351, write buffer="OUTP1:STAT OFF; :OUTP2:STAT OFF;") -> ()  [unwired: 1 in, 3 out]
                      n179 = Divide(x=w369, y=w357) -> (x/y=w364:dbl)
                      n180 = Divide(x=w361, y=w357) -> (x/y=w356:dbl)
                      n181 = Divide(x=w359, y=w357) -> (x/y=w355:dbl)
                      n182 = Divide(x=w368, y=w357) -> (x/y=w363:dbl)
                    }
                  }
                }
                frame #2 {
                  w387 = "\t"
                  # "Calculate contrast"
                  n183 = local read "Pulse mode"() -> (w378:T1)
                  n184 = Build Array (concatenate)(w395, w377) -> (w376:dbl[])
                  n185 = case shown="\"CW-ODMR\", Default" w378 {
                    tunnel: w377 -> [w402 w407 w412 w416]
                    tunnel: [w402 w406 w411 w415] -> w374
                    tunnel: w376 -> [w401 w405 w410 w417]
                    tunnel: [w401 w403 w408 w413] -> w375
                    frame "CW-ODMR", Default {
                    }
                    frame "Spin echo decay" {
                      w404 = 2.0 ("y")
                      n186 = Multiply(x=w407, y=w404) -> (x*y=w406:dbl)
                      n187 = Multiply(x=w405, y=w404) -> (x*y=w403:dbl[])
                    }
                    frame "Spin echo_IQ" {
                      w409 = 2.0 ("y")
                      n188 = Multiply(x=w412, y=w409) -> (x*y=w411:dbl)
                      n189 = Multiply(x=w410, y=w409) -> (x*y=w408:dbl[])
                    }
                    frame "XY8-N" {
                      n190 = local read "N of XY8-N"() -> (w418:i32)
                      n191 = expression code="x*16"(w418) -> (w414:i32)
                      n192 = Multiply(x=w416, y=w414) -> (x*y=w415:dbl)
                      n193 = Multiply(x=w417, y=w414) -> (x*y=w413:dbl[])
                    }
                  }
                  n194 = call "Convert to Dynamic Data"("Array"=w375) -> ("Dynamic Data Type"=w393:dynamicdata)  [unwired: 3 in]
                  n195 = case shown="\"sig1/ref2\"" "Contrast calculation" {
                    tunnel: w382 -> [w421 w424 w428 w433]
                    tunnel: w381 -> [w420 _ w429 w434]
                    tunnel: w380 -> [_ _ _ w431]
                    tunnel: w371 -> [_ w423 _ _]
                    tunnel: [w419 w422 w425 w430] -> w379
                    frame "sig1/sig2", Default {
                      n196 = Divide(x=w421, y=w420) -> (x/y=w419:dbl)
                    }
                    frame "sig1/ref2" {
                      n197 = Divide(x=w424, y=w423) -> (x/y=w422:dbl)
                    }
                    frame "(sig2-sig1)/(sig2+sig1)" {
                      n198 = Subtract(x=w429, y=w428) -> (x-y=w427:dbl)
                      n199 = Add(x=w429, y=w428) -> (x+y=w426:dbl)
                      n200 = Divide(x=w427, y=w426) -> (x/y=w425:dbl)
                    }
                    frame "(sig2-sig1)/ref1" {
                      n201 = Subtract(x=w434, y=w433) -> (x-y=w432:dbl)
                      n202 = Divide(x=w432, y=w431) -> (x/y=w430:dbl)
                    }
                  }
                  "Contrast" <- w379
                  n203 = Build Array (concatenate)(w396, w379) -> (w392:dbl[])
                  n204 = Format Into String(w390) -> (resulting string=w389:string)  [unwired: 3 in, 1 out]
                  n205 = Number To Fractional String(number=w379) -> (F-format string=w399:string)  [unwired: 3 in]
                  n206 = Number To Decimal String(number=w382) -> (decimal integer string=w398:string)  [unwired: 1 in]
                  n207 = Number To Decimal String(number=w380) -> (decimal integer string=w385:string)  [unwired: 1 in]
                  n208 = Number To Decimal String(number=w381) -> (decimal integer string=w386:string)  [unwired: 1 in]
                  n209 = Number To Decimal String(number=w371) -> (decimal integer string=w384:string)  [unwired: 1 in]
                  n210 = Number To Fractional String(number=w374, precision (6)=i16 1) -> (F-format string=w373:string)  [unwired: 2 in]
                  n211 = call "Convert to Dynamic Data2"("Array"=w392) -> ("Dynamic Data Type"=w391:dynamicdata)  [unwired: 3 in]
                  n212 = call "Build XY Graph"("Y Input"=w391, "X Input"=w393) -> ("XY Graph"=→"XY Graph":cluster{"X":dbl[], "Y":dbl[]}[])  [unwired: 8 in, 1 out]
                  n213 = Concatenate Strings(w389, w387, w373, w387, w399, w387, w398, w387, w385, w387, w386, w387, w384, "\r") -> (w400:string)
                  n214 = local read "file"() -> (w397:refnum<file>)
                  n215 = Write to Text File(file (use dialog)=w397, text=w400) -> ()  [unwired: 2 in, 3 out]
                  "Averaged counts" <- w371
                }
              }
              n216 = Greater Or Equal?(x=w179, y="Final duration (ns)") -> (x >= y?=w189:bool)
              n217 = local read "stop"() -> (w188:bool)
              n218 = Or(x=w189, y=w188) -> (x .or. y?=w187:bool)
            }
            n219 = Index Array(array=w170) -> (element=w168:dbl)  [unwired: 1 in]
            n220 = Build Array (concatenate)(w169, w168) -> (w167:dbl[])
          }
          frame #2 {
            # "Plot"
            n221 = call "Convert to Dynamic Data4"("Array"=w438) -> ("Dynamic Data Type"=w437:dynamicdata)  [unwired: 3 in]
            n222 = call "Convert to Dynamic Data3"("Array"=w436) -> ("Dynamic Data Type"=w435:dynamicdata)  [unwired: 3 in]
            n223 = call "Build XY Graph2"("Y Input"=w435, "X Input"=w437) -> ("XY Graph"=→"XY Graph 2":cluster{"X":dbl[], "Y":dbl[]}[])  [unwired: 8 in, 1 out]
          }
        }
        n224 = Greater Or Equal?(x=w159, y=w158) -> (x >= y?=w157:bool)
        n225 = Or(x=w157, y="stop") -> (x .or. y?=w155:bool)
      }
    }
    frame #3 {
      # "Instruments off"
      n226 = flat-sequence {
        tunnel: [w451] -> w440
        tunnel: w440 -> [w456]
        frame #0 {
          n227 = local read item#-1() -> (w446)
          n228 = VISA Close(VISA resource name=w446) -> ()  [unwired: 1 in, 1 out]
        }
        frame #1 {
          w447 = FALSE ("BNC output")
          n229 = local read "VISA_SG396"() -> (w448:refnum<visa-resource-name>)
          n230 = call "Set_SG394_Mode.vi"("Modulation"=w447, "N type output"=w447, "BNC output"=w447, "VISA resource name"=w448) -> ("VISA resource name out"=w449:refnum<visa-resource-name>)  [unwired: 6 in, 1 out]
          n231 = VISA Close(VISA resource name=w449) -> ()  [unwired: 1 in, 1 out]
        }
        frame #2 {
          w451 = dbl[unit] 0.01 ("Count Time Set")
          n232 = local read "VISA_SR400_2"() -> (w454:refnum<visa-resource-name>)
          n233 = call "SR400_settings_monitoring.vi"("Count Time Set"=w451, "# of periods (def: 1)"=1, "j (0)"=Output_Scale."Log", "Scan End Mode (Def: Stop)"=enum16{"Stop", "Start"}."Stop", "VISA_SR400"=w454) -> ("VISA resource name out"=w455:refnum<visa-resource-name>)
          n234 = VISA Close(VISA resource name=w455) -> ()  [unwired: 1 in, 1 out]
        }
        frame #3 {
          n235 = local read "VISA_SR400_1"() -> (w458:refnum<visa-resource-name>)
          n236 = call "SR400_settings_monitoring.vi"("Count Time Set"=w456, "# of periods (def: 1)"=1, "Scan End Mode (Def: Stop)"=enum16{"Stop", "Start"}."Stop", "VISA_SR400"=w458) -> ("VISA resource name out"=w457:refnum<visa-resource-name>)  [unwired: 1 in]
          n237 = VISA Close(VISA resource name=w457) -> ()  [unwired: 1 in, 1 out]
        }
      }
      n238 = local read "Location of spinapi.dll"() -> (w444:path)
      n239 = call "Laser_on_CW_pulse_sequence.vi"("Path"=w444) -> ("path out"=w445:path)
      n240 = call "Start_PulseBlaster.vi"("path in"=w445) -> ()  [unwired: 1 out]
      n241 = local read "Averaging?"() -> (w441:bool)
      n242 = case shown="False" w441 {
        frame False {
          n243 = local read "Measurement #"() -> (w461:i32)
          n244 = Increment(x=w461) -> (x+1=w462:i32)
          n245 = local write "Measurement #"(w462) -> ()
        }
        frame True {
        }
      }
      n246 = local read "file"() -> (w443:refnum<file>)
      n247 = Close File(refnum=w443) -> ()  [unwired: 1 in, 2 out]
      n248 = local write "stop"(FALSE ("Stop tracking")) -> ()
    }
  }
